vi "GetScanFormats.vi"(8 "ErrorIn(No Error)":errorcluster caption="entrée d'erreur (pas d'erreur)", 11 "Scan(T)":bool) -> (0 "sortie d'erreur":errorcluster, 2 "Cluster":T1, 3 "Prefixe":string)   [LabVIEW 2019]
uses:
  <vilib>/Utility/config.llb/Read Key (String).vi
  <vilib>/Utility/config.llb/Read Key (Boolean).vi
  <vilib>/Utility/config.llb/NI_LVConfig.lvlib
panel:
  in  "DisplayName":string caption="Prefixe"
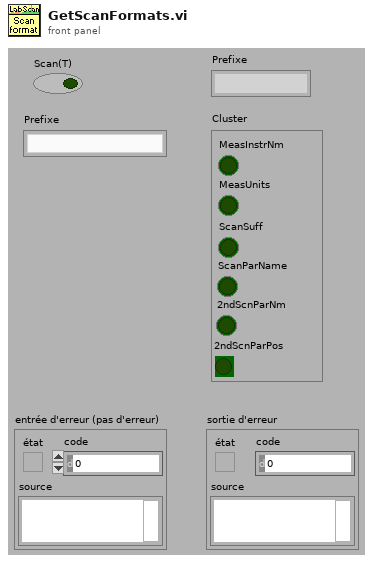
[diagram p1: front panel]
types:
  T1 = cluster{"MeasInstrNm":bool, "MeasUnits":bool, "ScanSuff":bool, "ScanParNm":bool, "2ndScnParNm":bool, "2ndScnParPos":bool}
  T2 = typedef "NI_LVConfig.lvlib/Config Data RefNum.ctl" = refnum<k1>
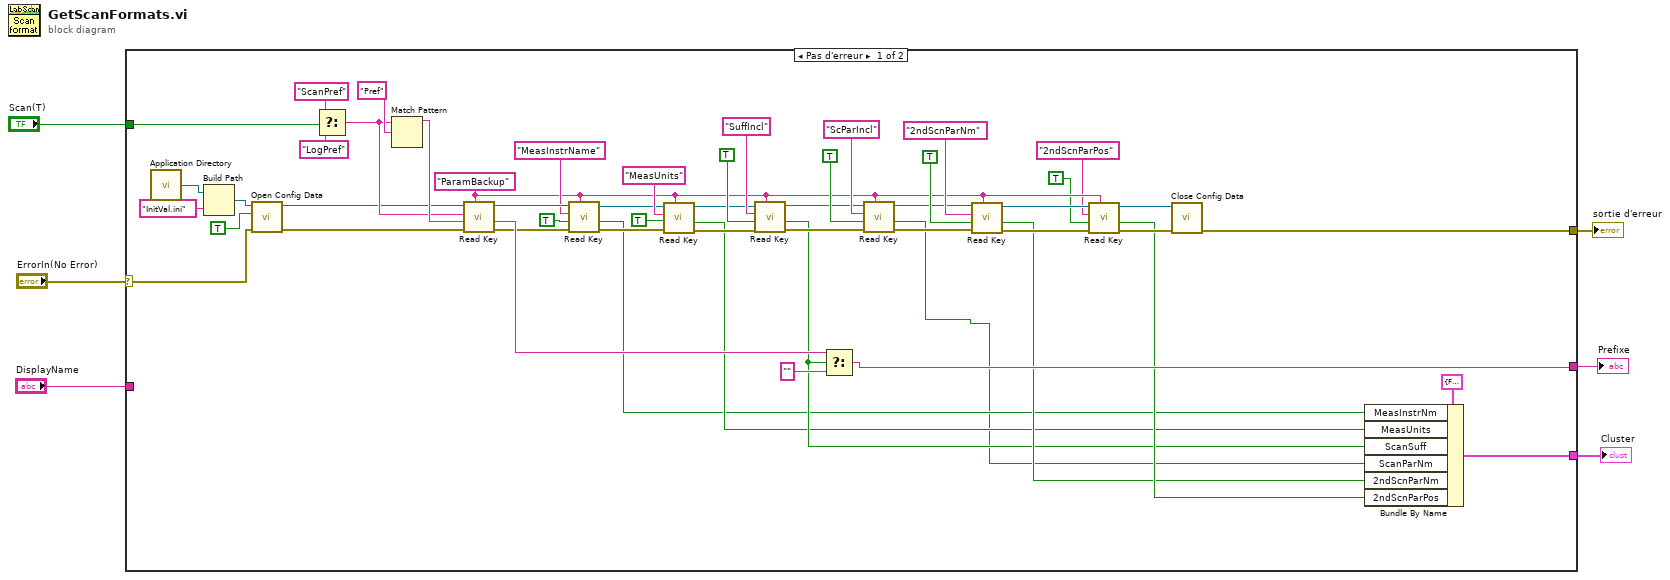
[diagram p0: block diagram]
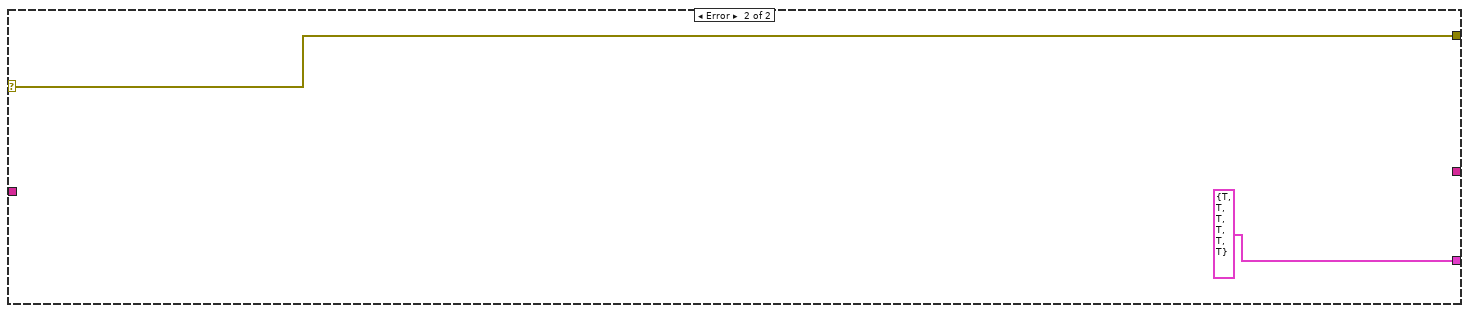
[diagram p2: hidden frame]
diagram:
  n1 = case shown="Pas d'erreur" "ErrorIn(No Error)" {
    selector: "ErrorIn(No Error)" -> [w47 w60]
    tunnel: [w46 w60] -> w5
    tunnel: "Scan(T)" -> [w43 _]
    tunnel: [w32 _] -> w3
    tunnel: "DisplayName" -> [_ _]
    tunnel: [w15 T1 {"MeasInstrNm"=TRUE, "MeasUnits"=TRUE, "ScanSuff"=TRUE, "ScanParNm"=TRUE, "2ndScnParNm"=TRUE, "2ndScnParPos"=TRUE} ("Cluster")] -> w1
    frame No Error {
      w17 = "ParamBackup"
      n2 = call <vilib>:"Application Directory.vi"() -> ("Application Directory"=w51:path)
      n3 = Build Path(base path=w51, name or relative path="InitVal.ini") -> (appended path=w50:path)
      n4 = call <vilib>:"Open Config Data.vi"("error in (no error)"=w47, "create file if necessary (T)"=TRUE ("create file if necessary? (T)"), "configuration file path"=w50) -> ("error out"=w52:errorcluster, "refnum"=w55:T2)  [unwired: 6 in, 1 out]
      n5 = Select(t="ScanPref", s=w43, f="LogPref") -> (s? t:f=w56:string)
      n6 = Match Pattern(string=w56, regular expression="Pref") -> (before substring=w58:string)  [unwired: 1 in, 3 out]
      n7 = call-poly <vilib>:"Read Key.vi"("section"=w17, "error in (no error)"=w52, "default value"=w58, "key"=w56, "refnum"=w55) -> ("error out"=w31:errorcluster, "value"=w34:string, "refnum out"=w30:T2)  [unwired: 3 in, 1 out]
      n8 = call-poly <vilib>:"Read Key.vi"("section"=w17, "error in (no error)"=w31, "default value"=TRUE, "key"="MeasInstrName", "refnum"=w30) -> ("error out"=w26:errorcluster, "value"=w9:bool, "refnum out"=w23:T2)  [unwired: 3 in, 1 out]
      n9 = call-poly <vilib>:"Read Key.vi"("section"=w17, "error in (no error)"=w26, "default value"=TRUE, "key"="MeasUnits", "refnum"=w23) -> ("error out"=w25:errorcluster, "value"=w10:bool, "refnum out"=w22:T2)  [unwired: 3 in, 1 out]
      n10 = call-poly <vilib>:"Read Key.vi"("section"=w17, "error in (no error)"=w25, "default value"=TRUE, "key"="SuffIncl", "refnum"=w22) -> ("error out"=w35:errorcluster, "value"=w11:bool, "refnum out"=w36:T2)  [unwired: 3 in, 1 out]
      n11 = Select(t=w34, s=w11, f="" ("cas faux")) -> (s? t:f=w32:string)
      n12 = call-poly <vilib>:"Read Key.vi"("section"=w17, "error in (no error)"=w35, "default value"=TRUE, "key"="ScParIncl", "refnum"=w36) -> ("error out"=w40:errorcluster, "value"=w8:bool, "refnum out"=w39:T2)  [unwired: 3 in, 1 out]
      n13 = call-poly <vilib>:"Read Key.vi"("section"=w17, "error in (no error)"=w40, "default value"=TRUE, "key"="2ndScnParNm", "refnum"=w39) -> ("error out"=w21:errorcluster, "value"=w12:bool, "refnum out"=w19:T2)  [unwired: 3 in, 1 out]
      n14 = call-poly <vilib>:"Read Key.vi"("section"=w17, "error in (no error)"=w21, "default value"=TRUE, "key"="2ndScnParPos", "refnum"=w19) -> ("error out"=w20:errorcluster, "value"=w13:bool, "refnum out"=w18:T2)  [unwired: 3 in, 1 out]
      n15 = call <vilib>:"Close Config Data.vi"("error in (no error)"=w20, "refnum"=w18) -> ("error out"=w46:errorcluster)  [unwired: 8 in, 1 out]
      n16 = Bundle By Name(cluster=T1 {"MeasInstrNm"=FALSE, "MeasUnits"=FALSE, "ScanSuff"=FALSE, "ScanParNm"=FALSE, "2ndScnParNm"=FALSE, "2ndScnParPos"=FALSE} ("Cluster"), "MeasInstrNm"=w9, "MeasUnits"=w10, "ScanSuff"=w11, "ScanParNm"=w8, "2ndScnParNm"=w12, "2ndScnParPos"=w13) -> (w15:T1)
    }
    frame Error {
    }
  }
  "sortie d'erreur" <- w5
  "Prefixe" <- w3
  "Cluster" <- w1
